vi "Teleop.vi"(10 "Match Info":T1={"Autonomous Elapsed Seconds"=0.0, "TeleOp Elapsed Seconds"=0.0, "Disabled Elapsed Seconds"=0.0, "Visited Autonomous"=FALSE, "Visited TeleOp"=FALSE, "Visited Disabled"=FALSE, "Autonomous Settings"={"Autonomous Style"=enum."Independent", "VI Refnum"=refnum}}, 11 "Call Context":T2) -> ()   [LabVIEW 2014]
doc: "This VI is called for each TeleOp packet received from the DS where the robot is not disabled. It is often used to read from the joysticks and update I/O or to update setpoints for timed control loops. It should complete and return within 20 milliseconds or it may miss DS packets."
uses:
  <vilib>/Rock Robotics/WPI/DriverStation/WPI_DriverStationDerivedRobotMode.ctl
  <vilib>/Rock Robotics/WPI/DriverStation/WPI_DriverStationMatch Info.ctl
  <vilib>/Rock Robotics/WPI/RobotDrive/WPI_RobotDriveGetSetRefNum.vi
  <vilib>/Rock Robotics/WPI/Joystick/WPI_JoystickGetSetRefNum.vi
  <vilib>/Rock Robotics/Network Tables/SD Write Boolean Array.vi
  <vilib>/Rock Robotics/Network Tables/SD Write Numeric Array.vi
  <vilib>/Rock Robotics/Network Tables/SD Read Boolean.vi
  <vilib>/Rock Robotics/Network Tables/SD Read Number.vi
  2015 Master Code RECYCLE RUSH/Modules 2015/Desired Arm Position.vi
  Robot Global Data.vi
panel:
  out "x+y":dbl
  out "Pusher Out":bool
  out "Front Arm Bottom":bool
  out "Front Arm Top":bool
  out "Sample Slider 0":dbl(slide) scale=0.0..5.0
  out "Sample Boolean 1":bool
  out "Sample Boolean 0":bool
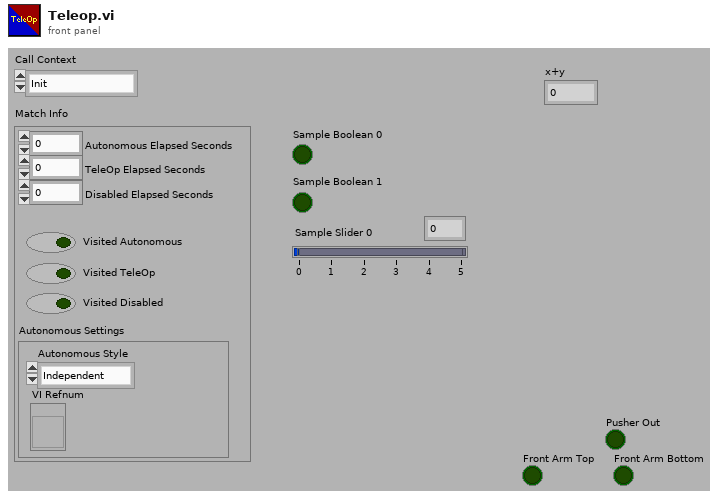
[diagram p1: front panel]
types:
  T1 = typedef "WPI_DriverStationMatch Info.ctl" = cluster{"Autonomous Elapsed Seconds":dbl, "TeleOp Elapsed Seconds":dbl, "Disabled Elapsed Seconds":dbl, "Visited Autonomous":bool, "Visited TeleOp":bool, "Visited Disabled":bool, "Autonomous Settings":cluster{"Autonomous Style":enum16{"Iterative", "Independent"}, "VI Refnum":refnum<vi>}}
  T2 = typedef "WPI_DriverStationDerivedRobotMode.ctl" = enum16{"Init", "Execute", "Stop"}
  T3 = typedef "WPI_JoystickDevRef.ctl" = cluster{"Device":T4}
  T4 = typedef "WPI_JoystickDeviceEnum.ctl" = enum16{"USB 0", "USB 1", "USB 2", "USB 3", "USB 4", "USB 5"}
  T5 = typedef "WPI_RobotDriveDevRef.ctl" = cluster{"DevStatus":errorcluster, "Motors[]":T6[], "Square Inputs":bool, "Max Output":dbl}
  T6 = typedef "WPI_MotorControlDeviceRef.ctl" = cluster{"DeviceStatus":errorcluster, "Type":T7, "PWM":cluster{"Controller":T8, "PWM Channel":T9, "DeadBand":T10}, "CAN":cluster{"Device Number":u8, "Control Mode":T11, "Semaphore":T12, "Max Vout":dbl, "TalonSRX Control Mode":T13}, "Invert":bool, "TransformRef":T14, "InvTransformRef":T14}
  T7 = typedef "WPI_MotorControlType.ctl" = enum16{"PWM", "CAN", "CANTalonSRX"}
  T8 = typedef "FPGA_TypedefDigitalModule.ctl" = enum16{"Controller 1"}
  T9 = typedef "FPGA_DIOPWMChannel.ctl" = enum8{"PWM 0", "PWM 1", "PWM 2", "PWM 3", "PWM 4", "PWM 5", "PWM 6", "PWM 7", "PWM 8", "PWM 9", "PWM MXP 0", "PWM MXP 1", "PWM MXP 2", "PWM MXP 3", "PWM MXP 4", "PWM MXP 5", "PWM MXP 6", "PWM MXP 7", "PWM MXP 8", "PWM MXP 9", "Invalid"}
  T10 = typedef "WPI_PWMDeadband.ctl" = cluster{"Name":string, "maxPositivePwm":i32, "minPositivePwm":i32, "centerPwm":i32, "maxNegativePwm":i32, "minNegativePwm":i32, "angularRange":u16}
  T11 = typedef "WPI_CANJaguar_ControlMode.ctl" = enum8{"Percent VBus", "Current", "Speed", "Position", "Voltage"}
  T12 = typedef "Semaphore RefNum" = refnum<k1>
  T13 = typedef "WPI_CANTalonSRX_APIControlMode.ctl" = enum8{"Percent VBus", "Speed", "Position", "Slave", "Unchanged / Invalid"}
  T14 = typedef "WPI_PWMTransform_ConPane.ctl" = refnum<vi>
  T15 = typedef "WPI_DigitalInputDevRef.ctl" = cluster{"DevStatus":errorcluster, "DIO Channel":T16, "Controller":T8}
  T16 = typedef "FPGA_DIOChannel.ctl" = enum8{"DIO 0", "DIO 1", "DIO 2", "DIO 3", "DIO 4", "DIO 5", "DIO 6", "DIO 7", "DIO 8", "DIO 9", "DIO MXP 0", "DIO MXP 1", "DIO MXP 2", "DIO MXP 3", "DIO MXP 4", "DIO MXP 5", "DIO MXP 6", "DIO MXP 7", "DIO MXP 8", "DIO MXP 9", "DIO MXP 10", "DIO MXP 11", "DIO MXP 12", "DIO MXP 13", "DIO MXP 14", "DIO MXP 15", "Invalid"}
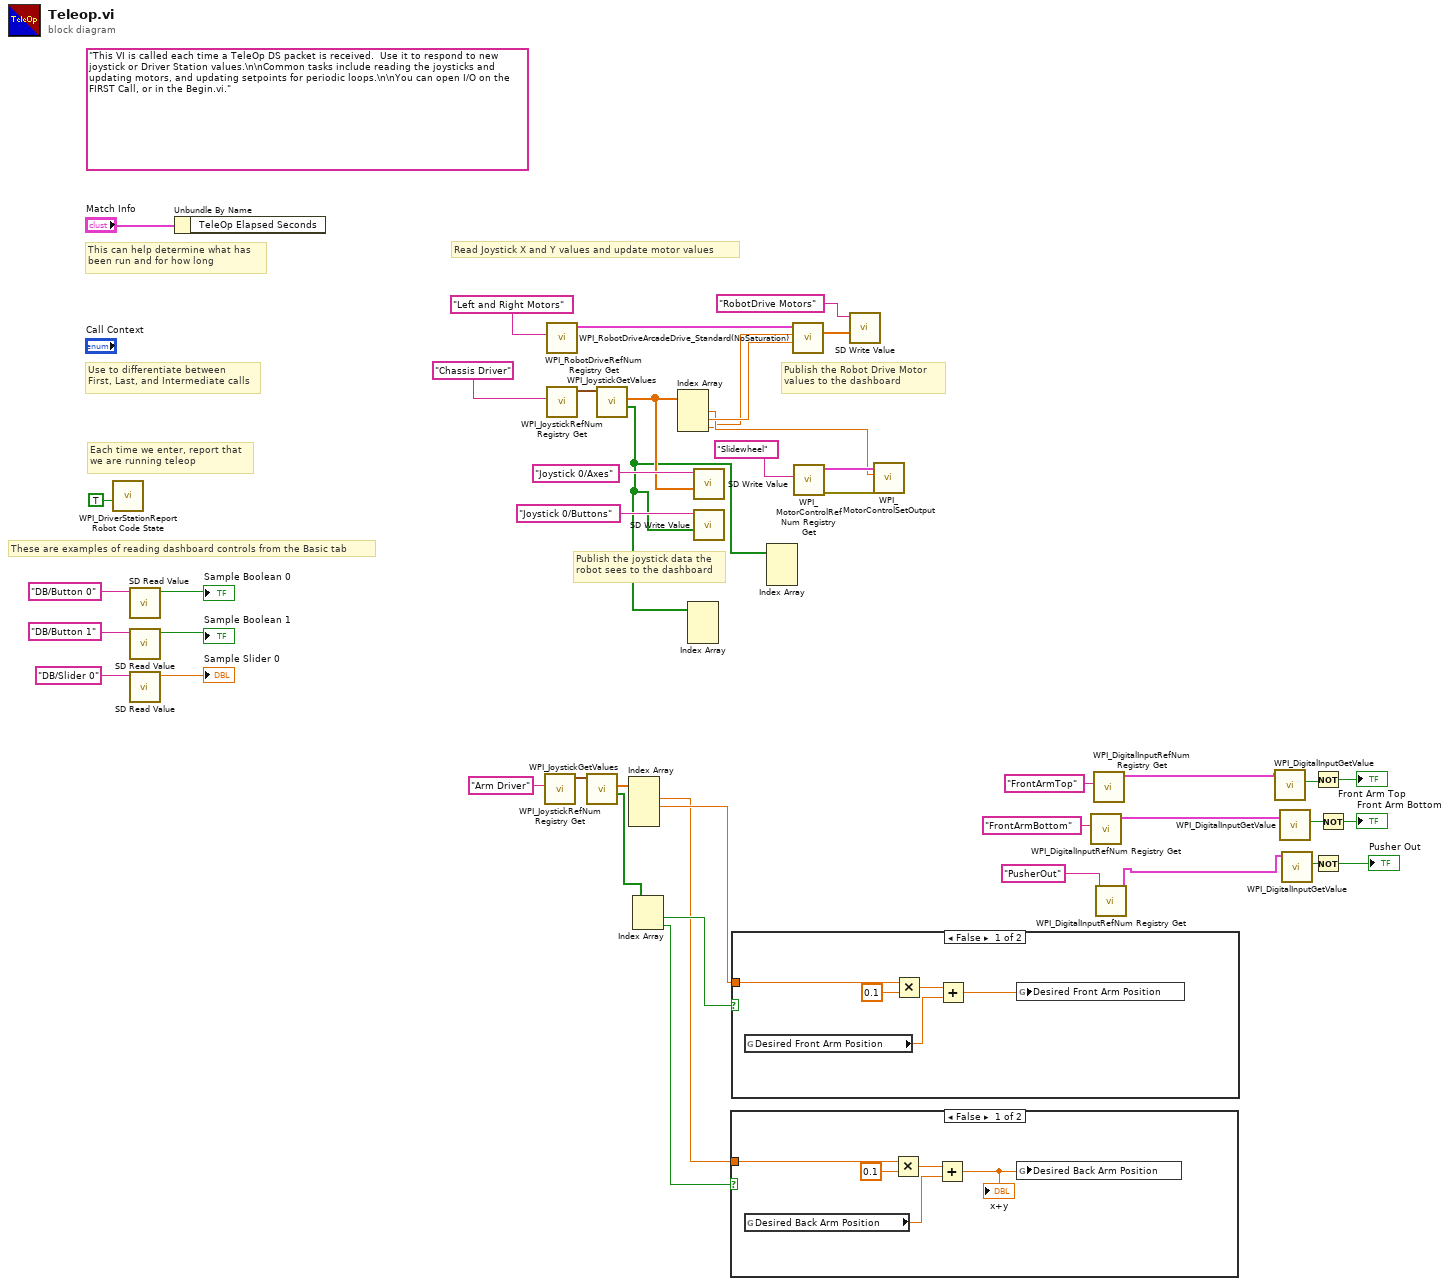
[diagram p0: block diagram]
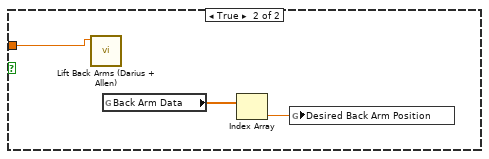
[diagram p2: hidden frame]
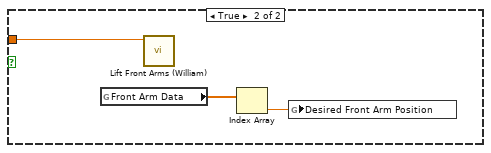
[diagram p3: hidden frame]
diagram:
  (unwired) "This VI is called each time a TeleOp DS packet is received.  Use it to respond to new joystick or Driver Station values.\n\nCommon tasks include reading the joysticks and updating motors, and updating setpoints for periodic loops.\n\nYou can open I/O on the FIRST Call, or in the Begin.vi."
  # "These are examples of reading dashboard controls from the Basic tab"
  # "Publish the Robot Drive Motor\nvalues to the dashboard"
  # "Publish the joystick data the\nrobot sees to the dashboard"
  # "Each time we enter, report that\nwe are running teleop"
  # "Use to differentiate between\nFirst, Last, and Intermediate calls"
  # "This can help determine what has\nbeen run and for how long"
  # "Read Joystick X and Y values and update motor values"
  n1 = call <vilib>:"WPI_DriverStationReport Robot Code State.vi"("TeleOp"=TRUE ("Autonomous")) -> ()  [unwired: 10 in, 1 out]
  n2 = call-poly <vilib>:"SD Read Value.vi"("Name"="DB/Button 0" ("refnum name")) -> ("Boolean"=→"Sample Boolean 0":bool)  [unwired: 8 in, 2 out]
  n3 = call-poly <vilib>:"SD Read Value.vi"("Name"="DB/Button 1" ("refnum name")) -> ("Boolean"=→"Sample Boolean 1":bool)  [unwired: 8 in, 2 out]
  n4 = call-poly <vilib>:"SD Read Value.vi"("Name"="DB/Slider 0" ("refnum name")) -> ("Numeric"=→"Sample Slider 0":dbl)  [unwired: 8 in, 2 out]
  n5 = Unbundle By Name("Match Info") -> ()  [unwired: 1 out]
  n6 = call <vilib>:"WPI_JoystickRefNum Registry Get.vi"("refnum name"="Arm Driver") -> ("JoystickDevRef"=w21:T3)  [unwired: 1 in, 9 out]
  n7 = call <vilib>:"WPI_RobotDriveRefNum Registry Get.vi"("refnum name"="Left and Right Motors") -> ("RobotDriveDevRef"=w42:T5)  [unwired: 1 in, 9 out]
  n8 = call <vilib>:"WPI_JoystickRefNum Registry Get.vi"("refnum name"="Chassis Driver") -> ("JoystickDevRef"=w40:T3)  [unwired: 1 in, 9 out]
  n9 = call <vilib>:"WPI_JoystickGetValues.vi"("JoystickDevRef"=w21) -> ("Buttons"=w5:bool[], "Axes"=w20:dbl[])  [unwired: 6 in, 3 out]
  n10 = call <vilib>:"WPI_JoystickGetValues.vi"("JoystickDevRef"=w40) -> ("Buttons"=w23:bool[], "Axes"=w28:dbl[])  [unwired: 6 in, 3 out]
  n11 = Index Array(array=w20) -> (element #1=w1:dbl, element #2=w2:dbl)  [unwired: 4 in, 2 out]
  n12 = Index Array(array=w5) -> (element #1=w4:bool, element #2=w3:bool)  [unwired: 2 in]
  n13 = Index Array(array=w28) -> (element #1=w7:dbl, element #2=w31:dbl, element #3=w6:dbl)  [unwired: 3 in]
  n14 = Index Array(array=w23) -> ()  [unwired: 3 in, 3 out]
  n15 = call-poly <vilib>:"SD Write Value.vi"("Numeric Array"=w28, "Name"="Joystick 0/Axes") -> ()  [unwired: 8 in, 2 out]
  n16 = call-poly <vilib>:"SD Write Value.vi"("Boolean Array"=w23, "Name"="Joystick 0/Buttons") -> ()  [unwired: 8 in, 2 out]
  n17 = case shown="False" w3 {
    tunnel: w1 -> [w49 w50]
    frame False {
      n18 = global read "Desired Arm Position.vi" "Desired Back Arm Position"() -> (w46:dbl)
      n19 = Multiply(x=w49, y=0.1) -> (x*y=w47:dbl)
      n20 = Add(x=w47, y=w46) -> (x+y=w45:dbl)
      "x+y" <- w45
      n21 = global write "Desired Arm Position.vi" "Desired Back Arm Position"(w45) -> ()
    }
    frame True {
      n22 = call "Lift Back Arms (Darius + Allen).vi"("Motor Output"=w50) -> ()  [unwired: 9 in, 2 out]
      n23 = global read "Robot Global Data.vi" "Back Arm Data"() -> (w52:dbl[])
      n24 = Index Array(array=w52) -> (element=w51:dbl)  [unwired: 1 in]
      n25 = global write "Desired Arm Position.vi" "Desired Back Arm Position"(w51) -> ()
    }
  }
  n26 = case shown="False" w4 {
    tunnel: w2 -> [w57 w60]
    frame False {
      n27 = global read "Desired Arm Position.vi" "Desired Front Arm Position"() -> (w54:dbl)
      n28 = Multiply(x=w57, y=0.1) -> (x*y=w55:dbl)
      n29 = Add(x=w55, y=w54) -> (x+y=w53:dbl)
      n30 = global write "Desired Arm Position.vi" "Desired Front Arm Position"(w53) -> ()
    }
    frame True {
      n31 = global read "Robot Global Data.vi" "Front Arm Data"() -> (w59:dbl[])
      n32 = call "Lift Front Arms (William).vi"("Motor Output"=w60) -> ()  [unwired: 9 in, 2 out]
      n33 = Index Array(array=w59) -> (element=w58:dbl)  [unwired: 1 in]
      n34 = global write "Desired Arm Position.vi" "Desired Front Arm Position"(w58) -> ()
    }
  }
  n35 = Index Array(array=w23) -> ()  [unwired: 3 in, 3 out]
  n36 = call <vilib>:"WPI_RobotDriveArcadeDrive_Standard(NoSaturation).vi"("Y axis value"=w31, "X axis value"=w6, "RobotDriveDevRef"=w42) -> ("Motor Values"=w30:dbl[])  [unwired: 1 in, 7 out]
  n37 = call <vilib>:"WPI_MotorControlRefNum Registry Get.vi"("refnum name"="Slidewheel") -> ("error out"=w26:errorcluster, "MotorControlDevRef"=w25:T6)  [unwired: 9 in]
  n38 = call-poly <vilib>:"SD Write Value.vi"("Numeric Array"=w30, "Name"="RobotDrive Motors") -> ()  [unwired: 8 in, 2 out]
  n39 = call <vilib>:"WPI_MotorControlSetOutput.vi"("error in (no error)"=w26, "Output"=w7, "MotorControlDevRef"=w25) -> ()  [unwired: 6 in, 3 out]
  n40 = call <vilib>:"WPI_DigitalInputRefNum Registry Get.vi"("refnum name"="FrontArmBottom") -> ("DigitalInputDevRef"=w12:T15)  [unwired: 9 in, 1 out]
  n41 = call <vilib>:"WPI_DigitalInputRefNum Registry Get.vi"("refnum name"="FrontArmTop") -> ("DigitalInputDevRef"=w13:T15)  [unwired: 9 in, 1 out]
  n42 = call <vilib>:"WPI_DigitalInputRefNum Registry Get.vi"("refnum name"="PusherOut") -> ("DigitalInputDevRef"=w11:T15)  [unwired: 9 in, 1 out]
  n43 = call <vilib>:"WPI_DigitalInputGetValue.vi"("DigitalInputDevRef"=w13) -> ("Value"=w16:bool)  [unwired: 8 in, 2 out]
  n44 = call <vilib>:"WPI_DigitalInputGetValue.vi"("DigitalInputDevRef"=w12) -> ("Value"=w15:bool)  [unwired: 8 in, 2 out]
  n45 = call <vilib>:"WPI_DigitalInputGetValue.vi"("DigitalInputDevRef"=w11) -> ("Value"=w14:bool)  [unwired: 8 in, 2 out]
  n46 = Not(x=w16) -> (.not. x?=→"Front Arm Top":bool)
  n47 = Not(x=w14) -> (.not. x?=→"Pusher Out":bool)
  n48 = Not(x=w15) -> (.not. x?=→"Front Arm Bottom":bool)
